vi "Get Favorite Color.vi"(8 "error in (no error)":errorcluster, 11 "OLopez in":refnum<class "OLopez.lvclass">) -> (0 "error out":errorcluster, 2 "Color Box":u32(colorbox)=16748288, 3 "OLopez out":refnum<class "OLopez.lvclass">)   [LabVIEW 2024, in "OLopez.lvclass"]
uses:
  OLopez.lvclass
  OLopez.lvclass/OLopez.ctl
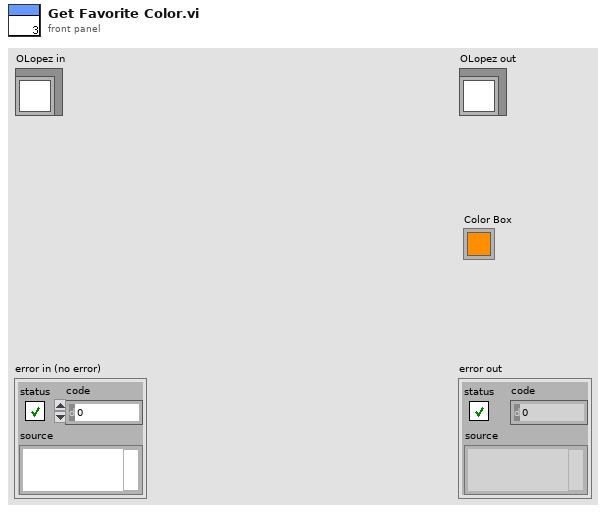
[diagram p1: front panel]
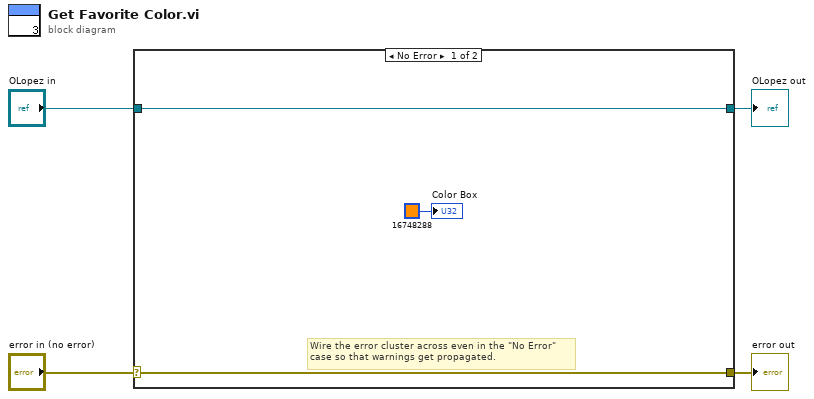
[diagram p0: block diagram]
diagram:
  n1 = case shown="No Error" "error in (no error)" {
    selector: "error in (no error)" -> [w6 w9]
    tunnel: [w6 w9] -> w3
    tunnel: [w7 w8] -> w1
    tunnel: "OLopez in" -> [w7 w8]
    frame No Error {
      # "Wire the error cluster across even in the \"No Error\"\ncase so that warnings get propagated."
      "Color Box" <- u32 16748288
    }
    frame Error {
    }
  }
  "error out" <- w3
  "OLopez out" <- w1
